vi "SLM 640 Set voltage.vi"(3 "Slave":u16[](array[numeric]), 4 "Master":u16[](array[numeric]), 5 "VISA Resource Name":refnum<visa-resource-name>="COM6") -> (0 "error out":errorcluster, 1 "Normal?":bool, 2 "dup VISA resource name":refnum<visa-resource-name>)   [LabVIEW 2022 SP3]
panel:
  out "Number of Pixels":u16
  in  "error in (no error)":errorcluster
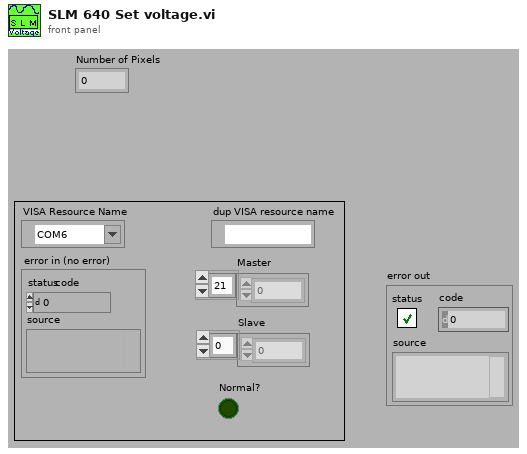
[diagram p1: front panel]
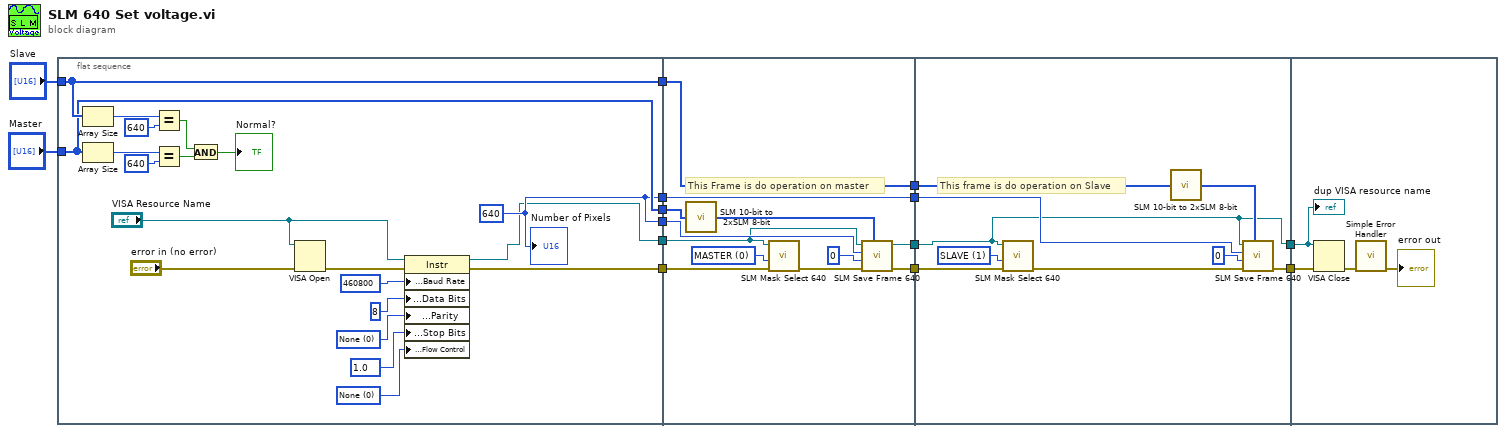
[diagram p0: block diagram]
diagram:
  n1 = flat-sequence {
    tunnel: [w16] -> w14
    tunnel: [w15] -> w13
    tunnel: [w17] -> w12
    tunnel: [w17] -> w9
    tunnel: [w21] -> w5
    tunnel: [w22] -> w3
    tunnel: "Slave" -> [w22]
    tunnel: "Master" -> [w21]
    tunnel: w14 -> [w35]
    tunnel: w13 -> [w41]
    tunnel: w12 -> [w46]
    tunnel: [w37] -> w11
    tunnel: [w36] -> w10
    tunnel: w9 -> [w45]
    tunnel: [w45] -> w8
    tunnel: w5 -> [w43]
    tunnel: [w42] -> w4
    tunnel: w3 -> [w42]
    tunnel: w11 -> [w47]
    tunnel: w10 -> [w52]
    tunnel: w8 -> [w55]
    tunnel: [w47] -> w7
    tunnel: [w48] -> w6
    tunnel: w4 -> [w53]
    tunnel: w7 -> [w59]
    tunnel: w6 -> [w58]
    frame #0 {
      w17 = 640
      w29 = u16 0 items=["None"=0, "XON/XOFF"=1, "RTS/CTS"=2, "DTR/DSR"=4] ("Serial Settings:Serial Flow Control")
      w30 = u16 10 items=["1.0"=10, "1.5"=15, "2.0"=20] ("Serial Settings:Serial Stop Bits")
      w31 = u16 0 items=["None", "Odd", "Even", "Mark", "Space"] ("Serial Settings:Serial Parity")
      n2 = Array Size(array=w22) -> (size(s)=w28:i32)
      n3 = Array Size(array=w21) -> (size(s)=w25:i32)
      n4 = Equal?(x=w28, y=640) -> (x = y?=w24:bool)
      n5 = Equal?(x=w25, y=640) -> (x = y?=w23:bool)
      n6 = And(x=w24, y=w23) -> (x .and. y?=→"Normal?":bool)
      n7 = VISA Open(error in (no error)="error in (no error)", VISA resource name="VISA Resource Name") -> (error out=w34:errorcluster)  [unwired: 3 in, 1 out]
      n8 = property class="Instr"(reference="VISA Resource Name", error in=w34, "Serial Settings:Baud Rate"=u32 460800 ("Serial Settings:Serial Baud Rate"), "Serial Settings:Data Bits"=u16 8 ("Serial Settings:Serial Data Bits"), "Serial Settings:Parity"=w31, "Serial Settings:Stop Bits"=w30, "Serial Settings:Flow Control"=w29) -> (reference out=w16:refnum<visa-resource-name>, error out=w15:errorcluster)
      "Number of Pixels" <- w17
    }
    frame #1 {
      w40 = u16 0 items=[" MASTER", " SLAVE"] ("MASTER or Slave mask?")
      # "This Frame is do operation on master"
      n9 = call "SLM 10-bit to 2xSLM 8-bit.vi"("Array of voltages"=w43) -> ("Array of SLM accepted voltages"=w44:u8[])
      n10 = call "SLM Mask Select 640.vi"("error in (no error)"=w41, "ACTIVE MASK"=w40, "VISA Resource Name"=w35) -> ("error out"=w39:errorcluster)  [unwired: 4 in]
      n11 = call "SLM Save Frame 640.vi"("Pixel Values"=w44, "error in (no error)"=w39, "Frame Number"=u32 0, "Number of Pixels"=w46, "VISA Resource Name"=w35) -> ("error out"=w36:errorcluster, "dup VISA resource name"=w37:refnum<visa-resource-name>)  [unwired: 2 in]
    }
    frame #2 {
      w50 = u16 1 items=[" MASTER", " SLAVE"] ("MASTER or Slave mask?")
      # "This frame is do operation on Slave"
      n12 = call "SLM Mask Select 640.vi"("error in (no error)"=w52, "ACTIVE MASK"=w50, "VISA Resource Name"=w47) -> ("error out"=w51:errorcluster)  [unwired: 4 in]
      n13 = call "SLM 10-bit to 2xSLM 8-bit.vi"("Array of voltages"=w53) -> ("Array of SLM accepted voltages"=w54:u8[])
      n14 = call "SLM Save Frame 640.vi"("Pixel Values"=w54, "error in (no error)"=w51, "Frame Number"=u32 0, "Number of Pixels"=w55, "VISA Resource Name"=w47) -> ("error out"=w48:errorcluster)  [unwired: 2 in, 1 out]
    }
    frame #3 {
      n15 = VISA Close(VISA resource name=w59, error in (no error)=w58) -> (error out=w57:errorcluster)
      n16 = call <vilib>:"Simple Error Handler.vi"("error in (no error)"=w57) -> ("error out"=→"error out":errorcluster)  [unwired: 4 in, 4 out]
      "dup VISA resource name" <- w59
    }
  }
